vi "Open vi Reference_2.2.0.0.vi"(4 "Close Front Panel(T)":bool, 5 "Wait Until Done":bool=TRUE, 6 "Front Panel State":T1(ring)=enum."Standard", 7 "Auto Dispose Reference":bool, 8 "error in":errorcluster, 10 "vi path":path) -> (0 "error out":errorcluster, 1 "VI Path":path, 2 "vi reference":refnum<vi>, 3 "hist_rev":string)   [LabVIEW 2018]
uses:
  <vilib>/Utility/error.llb/DialogType.ctl
  Sequence Globals.vi
panel:
  out "Stop Testing":bool
  in  "Front Panel Window:Is Frontmost":bool
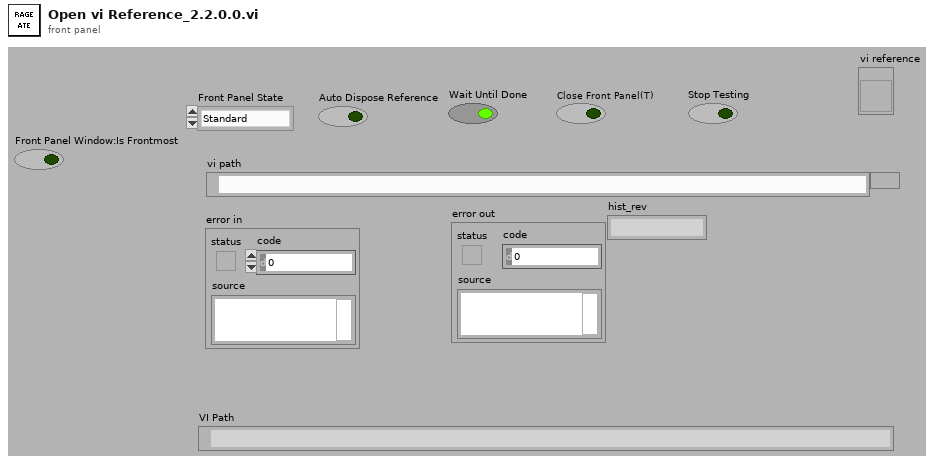
[diagram p1: front panel]
types:
  T1 = enum32{"Invalid", "Standard", "Closed", "Hidden", "Minimized", "Maximized"}
  T2 = typedef "DialogType.ctl" = u16
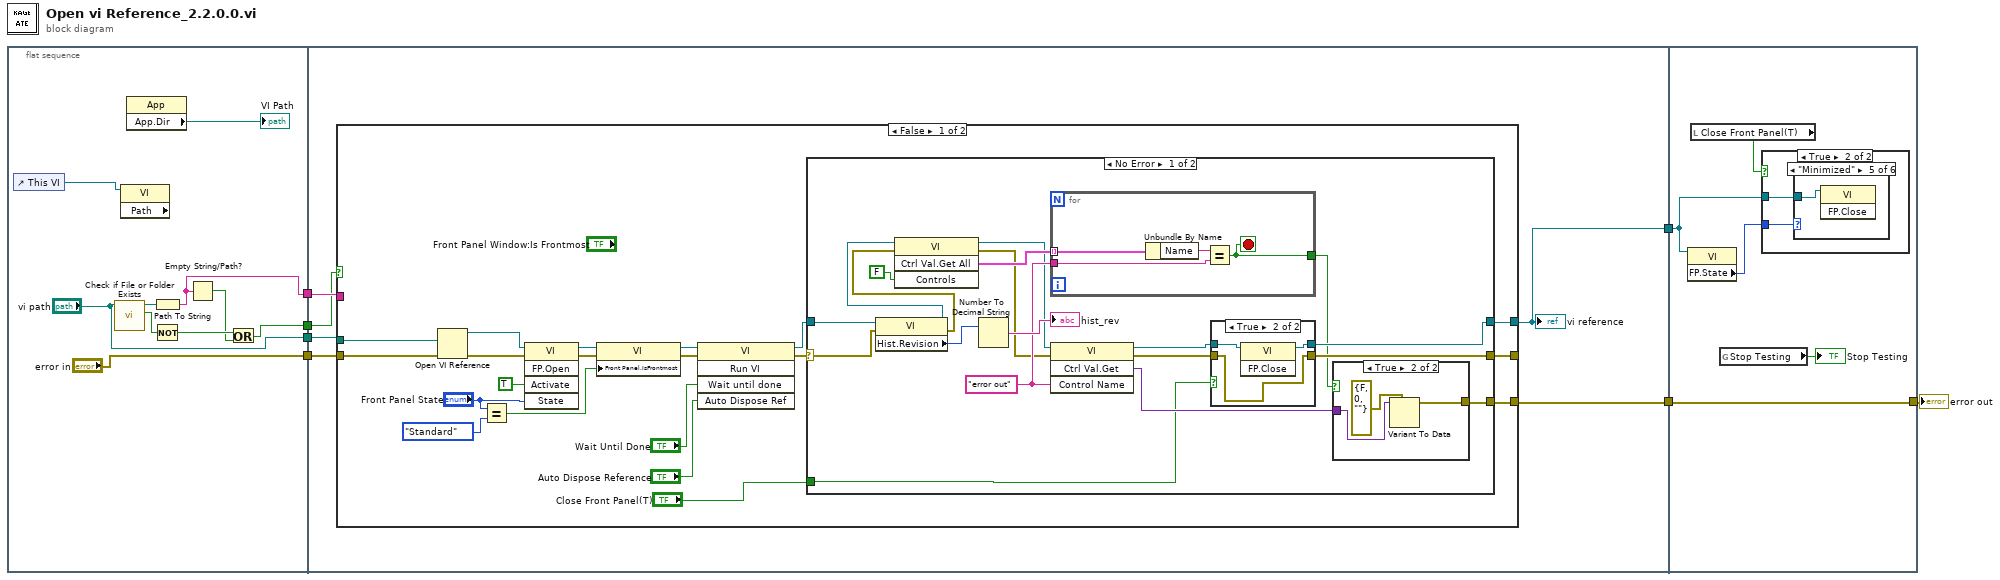
[diagram p0: block diagram]
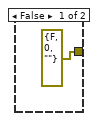
[diagram p2: hidden frame]
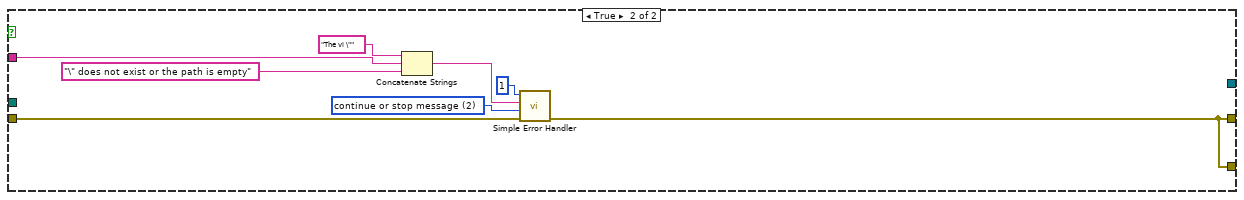
[diagram p5: hidden frame]
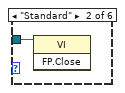
[diagram p8: hidden frame]
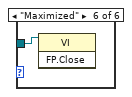
[diagram p11: hidden frame]
diagram:
  n1 = flat-sequence {
    tunnel: ["error in"] -> w4
    tunnel: ["vi path"] -> w3
    tunnel: [w12] -> w2
    tunnel: [w13] -> w1
    tunnel: [w19] -> w6
    tunnel: [w18] -> w5
    tunnel: w4 -> [w23]
    tunnel: w3 -> [w22]
    tunnel: w2 -> [w21]
    tunnel: w1 -> [w20]
    tunnel: [w90] -> w7
    tunnel: w6 -> [w87]
    tunnel: w5 -> [w90]
    frame #0 {
      n2 = control-ref of="This VI"() -> (w8:refnum<vi>)
      n3 = call <vilib>:"Check if File or Folder Exists.vi"("path"="vi path") -> ("file or folder exists?"=w15:bool, "dup path"=w14:path)  [unwired: 8 in, 1 out]
      n4 = property class="VI" props=["Path"](reference=w8) -> ()  [unwired: 1 in, 3 out]
      n5 = property class="App"() -> ("App.Dir"=→"VI Path":path)  [unwired: 2 in, 2 out]
      n6 = Path To String(path=w14) -> (string=w12:string)
      n7 = Not(x=w15) -> (.not. x?=w17:bool)
      n8 = Empty String/Path?(string/path=w12) -> (empty?=w16:bool)
      n9 = Or(x=w17, y=w16) -> (x .or. y?=w13:bool)
    }
    frame #1 {
      n10 = case shown="False" w20 {
        tunnel: [w43 _] -> w19
        tunnel: w22 -> [w42 _]
        tunnel: w23 -> [w38 w84]
        tunnel: [w37 w78] -> _
        tunnel: w21 -> [_ w79]
        tunnel: [w36 w78] -> w18
        frame False {
          n11 = Open VI Reference(vi path=w42, error in (no error)=w38) -> (vi reference=w33:refnum<vi>, error out=w29:errorcluster)  [unwired: 4 in]
          n12 = Equal?(x="Front Panel State", y=T1."Standard") -> (x = y?=w32:bool)
          n13 = invoke class="VI" method="FP.Open"(reference=w33, error in=w29, "Activate"=TRUE ("Activate FP?"), "State"="Front Panel State") -> (reference out=w26:refnum<vi>, error out=w28:errorcluster)  [unwired: 1 in, 3 out]
          n14 = property class="VI"(reference=w26, error in=w28, "Front Panel.IsFrontmost"=w32) -> (reference out=w25:refnum<vi>, error out=w27:errorcluster)
          n15 = invoke class="VI" method="Run VI"(reference=w25, error in=w27, "Wait until done"="Wait Until Done", "Auto Dispose Ref"="Auto Dispose Reference") -> (reference out=w35:refnum<vi>, error out=w34:errorcluster)  [unwired: 1 in, 3 out]
          n16 = case shown="No Error" w34 {
            selector: w34 -> [w49 w76]
            tunnel: [w62 w77] -> w43
            tunnel: [w61 w76] -> w37
            tunnel: [w59 w76] -> w36
            tunnel: w35 -> [w54 w77]
            tunnel: "Close Front Panel(T)" -> [w44 _]
            frame No Error {
              w51 = "error out" ("Control Name")
              n17 = property class="VI"(reference=w54, error in=w49) -> (reference out=w46:refnum<vi>, error out=w48:errorcluster, "Hist.Revision"=w56:u32)
              n18 = invoke class="VI" method="Ctrl Val.Get All"(reference=w46, error in=w48, "Controls"=FALSE) -> (reference out=w45:refnum<vi>, error out=w47:errorcluster, "Get All Control Values Variant"=w52:cluster{"Name":string, "Variant Data":variant}[])  [unwired: 1 in, 1 out]
              n19 = Number To Decimal String(number=w56) -> (decimal integer string=→"hist_rev":string)  [unwired: 1 in]
              n20 = for {
                tunnel: w52 -> [w70] mode=indexing
                tunnel: w51 -> [w68]
                tunnel: [w67] -> w50
                stop <- w67 stop-if-true
                n21 = Unbundle By Name(w70) -> ("Name"=w69:string)
                n22 = Equal?(x=w69, y=w68) -> (x = y?=w67:bool)
              }
              n23 = invoke class="VI" method="Ctrl Val.Get"(reference=w45, error in=w47, "Control Name"=w51) -> (reference out=w58:refnum<vi>, error out=w57:errorcluster, "Get Control Value Variant"=w60:variant)  [unwired: 1 in, 1 out]
              n24 = case shown="True" w44 {
                tunnel: [w72 w75] -> w62
                tunnel: w58 -> [w72 w74]
                tunnel: [w71 w73] -> w61
                tunnel: w57 -> [w71 w73]
                frame False {
                }
                frame True {
                  n25 = invoke class="VI" method="FP.Close"(reference=w74) -> (reference out=w75:refnum<vi>)  [unwired: 2 in, 2 out]
                }
              }
              n26 = case shown="True" w50 {
                tunnel: w60 -> [_ w66]
                tunnel: [errorcluster {"status"=FALSE, "code"=0, "source"=""} ("type") w64] -> w59
                frame False {
                }
                frame True {
                  n27 = Variant To Data(type=errorcluster {"status"=FALSE, "code"=0, "source"=""}, Variant=w66) -> (data=w64:errorcluster)  [unwired: 1 in, 1 out]
                }
              }
            }
            frame Error {
            }
          }
        }
        frame True {
          w85 = T2 2 items=["no dialog", "OK message", "continue or stop message", "OK message + warnings", "continue/stop + warnings"] ("type of dialog (OK msg:1)")
          n28 = Concatenate Strings("The vi \"", w79, "\" does not exist or the path is empty" ("string")) -> (w82:string)
          n29 = call <vilib>:"Simple Error Handler.vi"("error code (no error:0)"=1, "error source (\" \")"=w82, "type of dialog (OK msg:1)"=w85, "error in (no error)"=w84) -> ("error out"=w78:errorcluster)  [unwired: 1 in, 4 out]
        }
      }
      "vi reference" <- w19
    }
    frame #2 {
      n30 = property class="VI"(reference=w87) -> ("FP.State"=w88:T1)  [unwired: 1 in, 2 out]
      n31 = local read "Close Front Panel(T)"() -> (w89:bool)
      n32 = global read "Sequence Globals.vi" "Stop Testing"() -> (→"Stop Testing":bool)
      n33 = case shown="True" w89 {
        tunnel: w87 -> [_ w92]
        tunnel: w88 -> [_ w91]
        frame False {
        }
        frame True {
          n34 = case shown="\"Minimized\"" w91 {
            tunnel: w92 -> [_ w93 _ _ w94 w95]
            frame "Invalid", Default {
            }
            frame "Standard" {
              n35 = invoke class="VI" method="FP.Close"(reference=w93) -> ()  [unwired: 2 in, 3 out]
            }
            frame "Closed" {
            }
            frame "Hidden" {
            }
            frame "Minimized" {
              n36 = invoke class="VI" method="FP.Close"(reference=w94) -> ()  [unwired: 2 in, 3 out]
            }
            frame "Maximized" {
              n37 = invoke class="VI" method="FP.Close"(reference=w95) -> ()  [unwired: 2 in, 3 out]
            }
          }
        }
      }
    }
  }
  "error out" <- w7
